vi "Valid Guesses--constant.vi"() -> (2 "Valid Guesses (array)":string[](array[string]), 3 "Valid Guesses (set)":set{string}(c389))   [LabVIEW 2020]
doc: "All valid guesses for the Wordle word. The target word was selected from an undisclosed subset of the words in this list.\n\nNote that this VI returns the list as both an array of strings, and a set of strings."
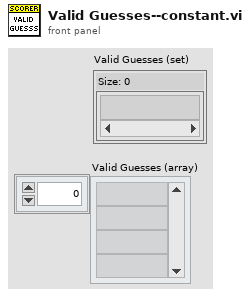
[diagram p1: front panel]
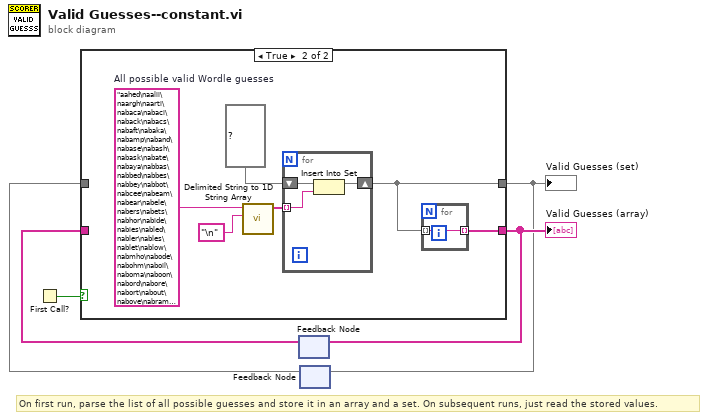
[diagram p0: block diagram]
diagram:
  # "On first run, parse the list of all possible guesses and store it in an array and a set. On subsequent runs, just read the stored values."
  n1 = First Call?() -> (First Call?: T/F=w1:bool)
  n2 = feedback #1() -> (w4:string[])  [unwired: 1 in]
  n3 = feedback #2() -> (w2:set{string})  [unwired: 1 in]
  n4 = case shown="True" w1 {
    tunnel: [w6 w13] -> w3
    tunnel: [w7 w12] -> w5
    tunnel: w4 -> [w7 _]
    tunnel: w2 -> [w6 _]
    frame False {
    }
    frame True {
      w11 = "aahed\naalii\naargh\naarti\nabaca\nabaci\naback\nabacs\nabaft\nabaka\nabamp\naband\nabase\nabash\nabask\nabate\nabaya\nabbas\nabbed\nabbes\nabbey\nabbot\nabcee\nabeam\nabear\nabele\nabers\nabets\nabhor\nabide\nabies\nabled\nabler\nables\nablet\nablow\nabmho\nabode\nabohm\naboil\naboma\naboon\nabord\nabore\nabort\nabout\nabove\nabram\nabray\nabrim\nabrin\nabris\nabsey\nabsit\nabuna\nabune\nabuse\nabuts\nabuzz\nabyes\nabysm\nabyss\nacais\nacari\naccas\naccoy\nacerb\nacers\naceta\nachar\nached\naches\nachoo\nacids\nacidy\nacing\nacini\nackee\nacker\nacmes\nacmic\nacned\nacnes\nacock\nacold\nacorn\nacred\nacres\nacrid\nacros\nacted\nactin\nacton\nactor\nacute\nacyls\nadage\nadapt\nadaws\nadays\n..."  # All possible valid Wordle guesses
      n5 = call <vilib>:"Delimited String to 1D String Array.vi"("delimiter"="\n", "delimited string"=w11) -> ("string array"=w10:string[])  [unwired: 9 in]
      n6 = for {
        tunnel: w10 -> [w14] mode=indexing
        shift-right: [w16] -> w13
        shift-left: set{string} {} ("Valid Guesses") -> [w15]
        n7 = Insert Into Set(10:w14, 11:w15) -> (3:w16:set{string})  [unwired: 1 out]
      }
      n8 = for {
        tunnel: [w17] -> w12 mode=indexing
        tunnel: w13 -> [w17] mode=indexing
      }
    }
  }
  "Valid Guesses (set)" <- w3
  "Valid Guesses (array)" <- w5
  n9 = feedback-in #1(w5) -> ()
  n10 = feedback-in #2(w3) -> ()
